vi "workbook.scope_type.vi"(8 "error in":errorcluster, 11 "Workbook in":refnum<class "Workbook.lvclass">) -> (0 "error out":errorcluster, 3 "Workbook out":refnum<class "Workbook.lvclass">)   [LabVIEW 2020, in "Workbook.lvclass"]
doc: "Returns whether the workbook's data scope is assets or runs."
uses:
  Workbook.lvclass
  client.lvlib
panel:
  out "out_type out":i32
  in  "out_type":i32
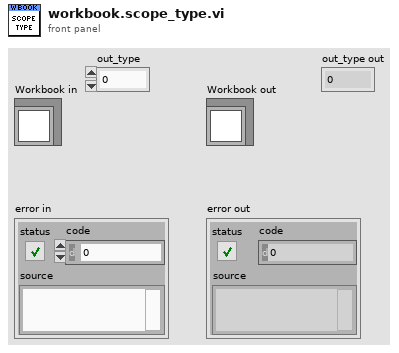
[diagram p1: front panel]
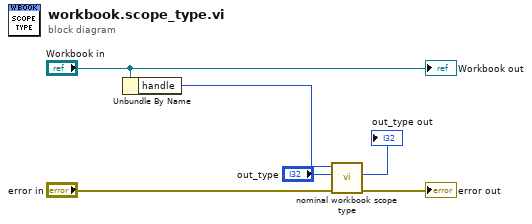
[diagram p0: block diagram]
diagram:
  n1 = Unbundle By Name("Workbook in") -> ("handle"=w4:i32)
  n2 = call "nominal workbook scope type.vi"("error in (no error)"="error in", "out_type"="out_type", "workbook"=w4) -> ("error out"=→"error out":errorcluster, "out_type out"=→"out_type out":i32)  [unwired: 6 in, 1 out]
  "Workbook out" <- "Workbook in"
